vi "L03.vi"() -> ()   [LabVIEW 2012]
panel:
  out "max value":i32
  out "Numeric":i32
  in  "x":i64=13195
  out "Array":i32[](array[numeric])
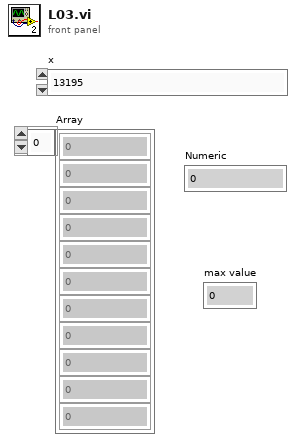
[diagram p1: front panel]
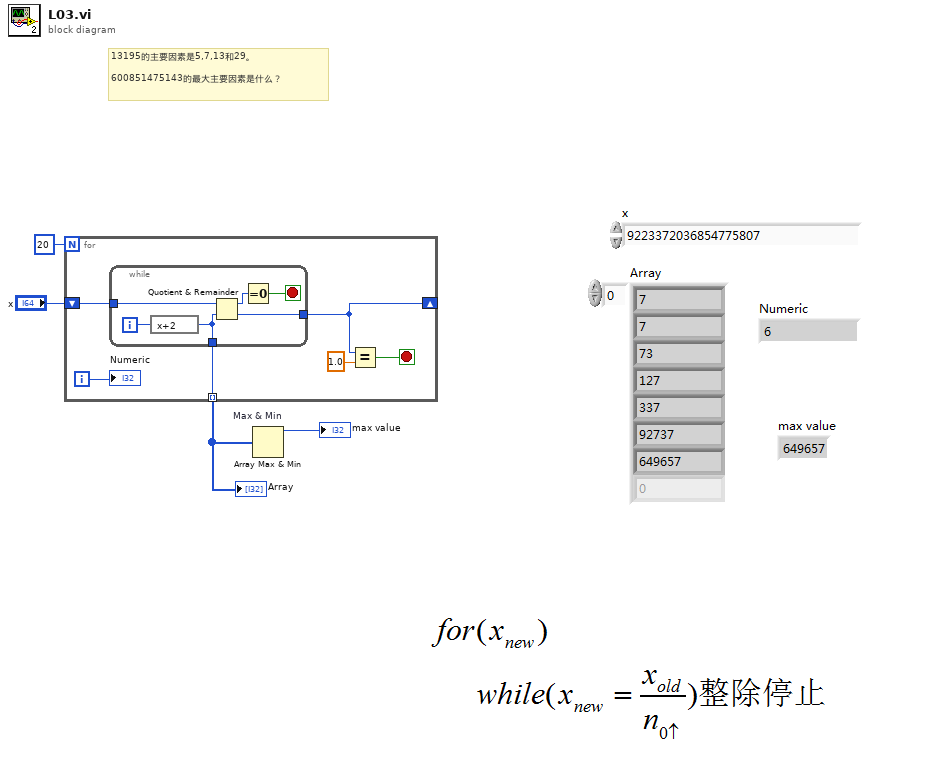
[diagram p0: block diagram]
diagram:
  # "13195的主要因素是5,7,13和29。\n\n600851475143的最大主要因素是什么？"
  n1 = for {
    N: 20 -> [_]
    shift-right: [w8] -> _
    shift-left: "x" -> [w10]
    tunnel: [w9] -> w2 mode=indexing
    i -> [w5]
    stop <- w6 stop-if-true
    n2 = while {
      tunnel: w10 -> [w16]
      tunnel: [w14] -> w8
      tunnel: [w11] -> w9
      i -> [w12]
      stop <- w13 stop-if-true
      n3 = expression code="x+2"(w12) -> (w11:i32)
      n4 = Quotient & Remainder(x=w16, y=w11) -> (x-y*floor(x/y)=w15:i64, floor(x/y)=w14:i64)
      n5 = Equal To 0?(x=w15) -> (x = 0?=w13:bool)
    }
    n6 = Equal?(x=w8, y=1.0) -> (x = y?=w6:bool)
    "Numeric" <- w5
  }
  "Array" <- w2
  n7 = Array Max & Min "Max & Min"(array=w2) -> (max value=→"max value":i32)  [unwired: 3 out]
